vi "Stop Core.vi"(10 "final error code":i32, 11 "Gui in":refnum<class "Gui.lvclass">) -> (3 "Gui out":refnum<class "Gui.lvclass">)   [LabVIEW 2022 SP3, in "Gui.lvlib" / "Gui.lvclass"]
doc: "(<B>Filename</B>: Actor Framework.lvlib:Actor.lvclass:Stop Core.vi)\n\nDefines what the actor does before it stops. Use the <B>final error code</B> input to determine whether the actor shut down in response to an error.\n\nBy default, this method does nothing. A descendant class may override it to define behavior, such as shutting down any processes the actor initiated in its override of the Actor Core method."
uses:
  Gui.lvclass
  Gui.lvclass/Gui.ctl
  LoggingActor/Source/LoggingActor/LoggingActor/LoggingActor.lvclass
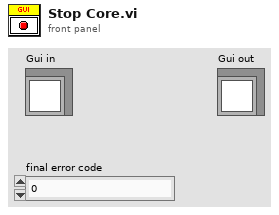
[diagram p1: front panel]
types:
  T1 = typedef "Gui.lvlib/Gui.lvclass/_Events.ctl" = cluster{"StopGuiLoop":refnum<user-event>}
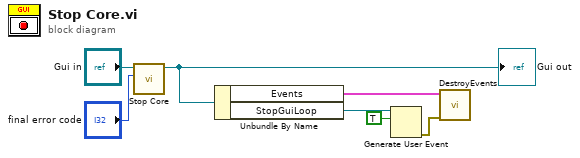
[diagram p0: block diagram]
diagram:
  n1 = call-parent "Stop Core.vi"("final error code"="final error code", "LoggingActor in"="Gui in") -> ("LoggingActor out"=w5:refnum<class "Gui.lvclass">)  [unwired: 9 in]
  "Gui out" <- w5
  n2 = Unbundle By Name(w5) -> ("Events"=w2:T1, "StopGuiLoop"=w4:refnum<user-event>)
  n3 = Generate User Event(user event=w4, event data cluster=TRUE ("event data")) -> (error out=w1:errorcluster)  [unwired: 2 in, 1 out]
  n4 = call "DestroyEvents.vi"("error in (no error)"=w1, "Events"=w2) -> ()  [unwired: 9 in, 1 out]
